vi "QR Get All Queues.vi"(8 "error in (no error)":errorcluster) -> (0 "error out":errorcluster, 1 "Number of Queues":i32, 2 "All Properties":T1[](array[typedef]), 3 "All Queues":T2[](array[typedef]))   [LabVIEW 2014, in "AMC.lvlib"]
doc: "This VI removes the host connection from the connection manager list if it becomes disconnected for any reason."
uses:
  AMC.lvlib
  _SubVIs/TypeDefs/Message Queue.ctl
  _SubVIs/TypeDefs/Message.ctl
  Keyed Array/KeyedArray.ctl
  _TypeDefs/QueueRegistryProperties.ctl
  _TypeDefs/QueueRegistryMethod.ctl
  Keyed Array/Tools_KeyedArray.lvlib
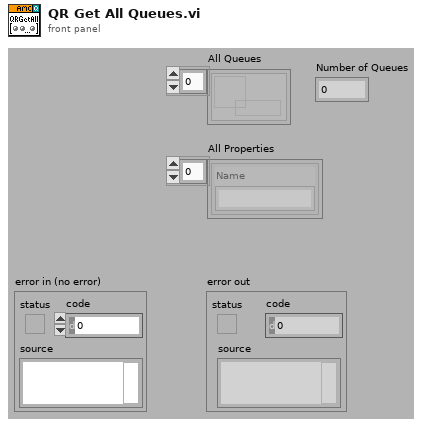
[diagram p1: front panel]
types:
  T1 = typedef "AMC.lvlib/QueueRegistryProperties.ctl" = cluster{"Name":string}
  T2 = typedef "AMC.lvlib/Message Queue.ctl" = refnum<queue>
  T3 = typedef "AMC.lvlib/QueueRegistryMethod.ctl" = enum16{"Initialize", "Add Queue", "Set Properties", "Get Queue by Index", "Get Queue by Name", "Remove Queue", "Remove All Queues"}
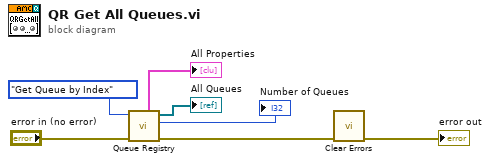
[diagram p0: block diagram]
diagram:
  n1 = call "Queue Registry.vi"("error in (no error)"="error in (no error)", "Method"=QueueRegistryMethod."Get Queue by Index") -> ("error out"=w5:errorcluster, "Number of Queues"=→"Number of Queues":i32, "All Queues"=→"All Queues":T2[], "All Properties"=→"All Properties":T1[])  [unwired: 3 in, 3 out]
  n2 = call <vilib>:"Clear Errors.vi"("error in (no error)"=w5) -> ("error out"=→"error out":errorcluster)  [unwired: 1 in, 5 out]
